vi "ziModGetNextNode.vi"(8 "Error In":errorcluster, 11 "ModHandle In":T5 {"ModHandle" format="0x%08x"; "Conn" format="0x%08x"}) -> (0 "Error Out":errorcluster, 2 "ModResults":T1, 3 "ModHandle Out":T5 {"ModHandle" format="0x%08x"; "Conn" format="0x%08x"}, 4 "NoData":bool)   [LabVIEW 2016, in "Zurich Instruments LabOne.lvlib"]
doc: "Use this device to extract the data from subscribed node, which you polled from device by ziModExecute.vi (with modal is false) or the ziModRead.vi. This allows to iterate through ModResults and return the <b>Path, the ValueType and the NoOfResults</b>. If this iterator, does not find any more data, the <b>NoData</b> flag is raised."
uses:
  Zurich Instruments LabOne.lvlib
  ziTypeModHandle.ctl
  ziTypeModResults.ctl
  Data/ziTypePollType.ctl
  ziTypeModSWTriggerHeader.ctl
  ziTypeModSweeperHeader.ctl
  ziModGetSWTriggerHeader.vi
  ziModGetSweeperHeader.vi
  Private/ziLV64.dll
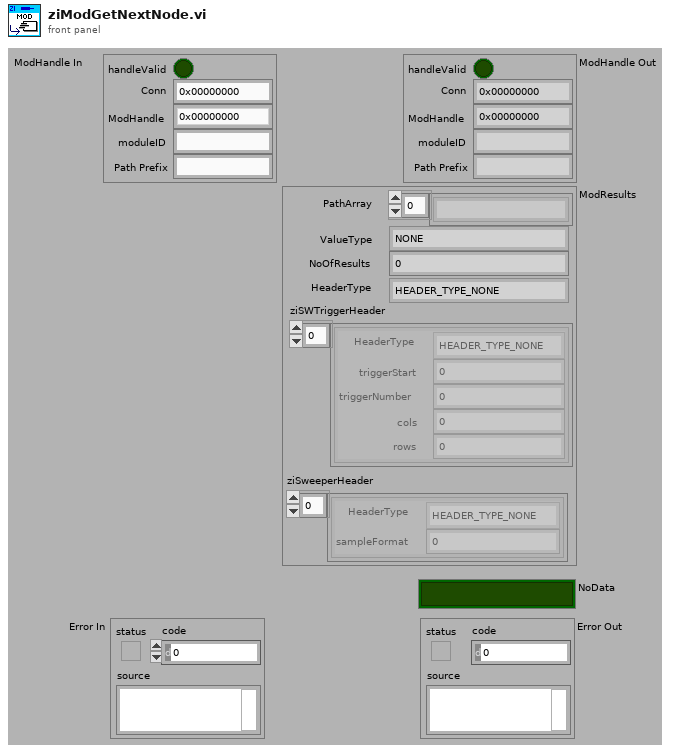
[diagram p1: front panel]
types:
  T1 = typedef "Zurich Instruments LabOne.lvlib/ziTypeModResults.ctl" = cluster{"PathArray":string[], "ValueType":T2, "NoOfResults":u64, "HeaderType":enum16{"HEADER_TYPE_NONE", "HEADER_TYPE_SWTRIGGER", "HEADER_TYPE_SWEEPER"}, "ziSWTriggerHeader":T3[], "ziSweeperHeader":T4[]}
  T2 = typedef "Zurich Instruments LabOne.lvlib/ziTypePollType.ctl" = enum16{"NONE", "DOUBLE_DATA", "INTEGER_DATA", "DEMOD_SAMPLE", "SCOPE_WAVE_HF2", "AUXIN_SAMPLE", "DIO_SAMPLE", "BYTE_ARRAY", "PWA_WAVE", "9", "10", "11", "12", "13", "14", "15", "TREE_CHANGE_DEPRI", "17", "ERROR", "19", "20", "21", "22", "23", "24", "25", "26", "27", "28", "29", "30", "31", "DOUBLE_DATA_TS", "INTEGER_DATA_TS", "34", "SCOPE_WAVE", "36", "37", "BYTE_ARRAY_TS", "39", "40", "41", "42", "43", "44", "45", "CNT_DATA", "47", "TREE_CHANGE", "49", "50", "51", "52", "53", "54", "55", "56", "57", "58", "59", "60", "61", "62", "63", "SWEEPER_DATA", "SPECTRUM_DATA", "ADVISOR_DATA", "67", "IMP_DATA"}
  T3 = typedef "Zurich Instruments LabOne.lvlib/ziTypeModSWTriggerHeader.ctl" = cluster{"HeaderType":enum8{"HEADER_TYPE_NONE", "HEADER_TYPE_SWTRIGGER", "HEADER_TYPE_SWEEPER"}, "triggerStart":u64, "triggerNumber":u64, "cols":u32, "rows":u32}
  T4 = typedef "Zurich Instruments LabOne.lvlib/ziTypeModSweeperHeader.ctl" = cluster{"HeaderType":enum8{"HEADER_TYPE_NONE", "HEADER_TYPE_SWTRIGGER", "HEADER_TYPE_SWEEPER"}, "sampleFormat":u8}
  T5 = typedef "Zurich Instruments LabOne.lvlib/ziTypeModHandle.ctl" = cluster{"handleValid":bool, "Conn":u64, "ModHandle":u64, "moduleID":string, "Path Prefix":string}
  T6 = enum16{"HEADER_TYPE_NONE", "HEADER_TYPE_SWTRIGGER", "HEADER_TYPE_SWEEPER"}
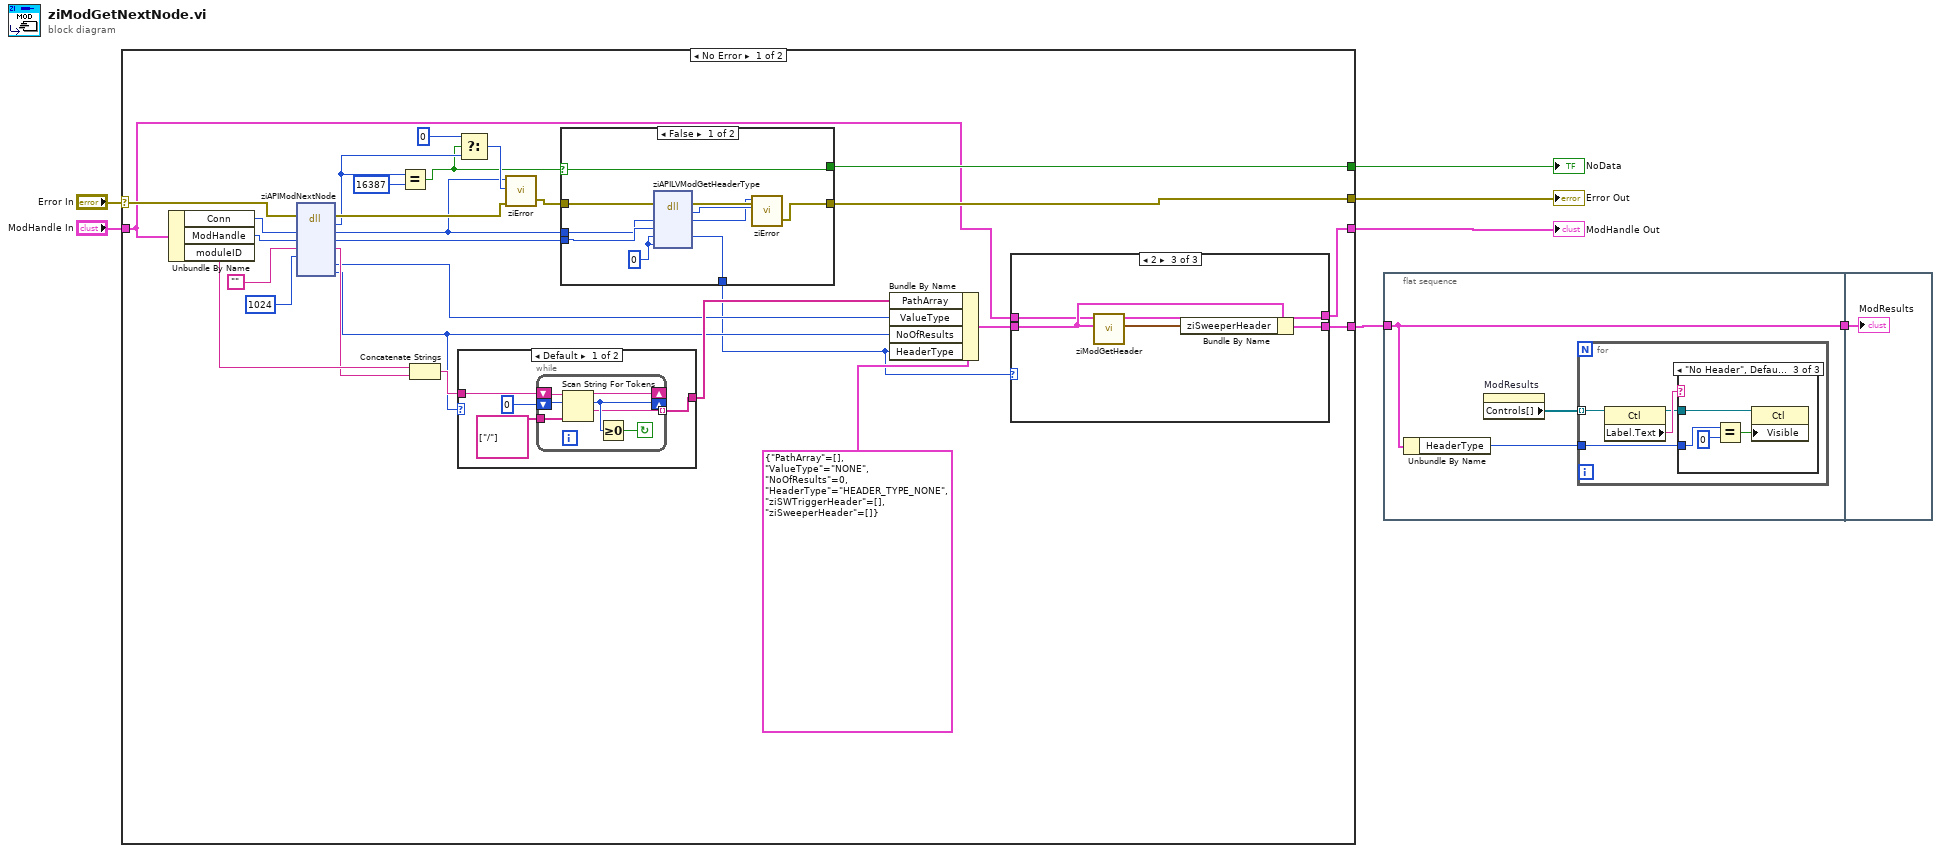
[diagram p0: block diagram]
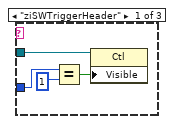
[diagram p2: hidden frame]
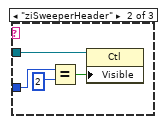
[diagram p3: hidden frame]
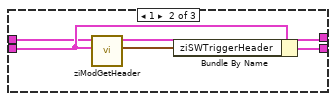
[diagram p5: hidden frame]
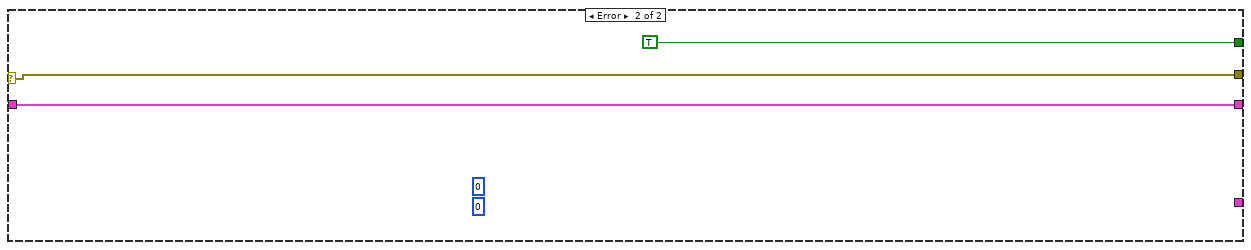
[diagram p8: hidden frame]
diagram:
  n1 = case shown="No Error" "Error In" {
    selector: "Error In" -> [w33 w71]
    tunnel: [w21 w71] -> w3
    tunnel: [w9 w73] -> w4
    tunnel: "ModHandle In" -> [w10 w73]
    tunnel: [w18 TRUE] -> w5
    tunnel: [w11 _] -> w2
    frame No Error {
      n2 = Unbundle By Name(w10) -> ("Conn"=w35:u64, "ModHandle"=w34:u64, "moduleID"=w25:string)
      n3 = dll-call lib="C:/Users/putkonen.CPFS/Desktop/resonant_ultrasound_arxiv/maglab ultrasound -- arkady --arxiv/Zurich/Zurich Instruments/LabOne/API/LabVIEW/Zurich Instruments LabOne/Private/ziLV*.*" fn="ziAPIModNextNode"(error in=w33, "Conn"=w35, "ModHandle"=w34, "Path"="", "bufferSize"=u32 1024) -> (error out=w32:errorcluster, "return type"=w28:u32, "Conn"=w17:u64, "ModHandle"=w22:u64, "Path"=w24:string, "valueType"=w14:u64, "NoOfResults"=w15:u64)  [unwired: 5 in, 1 out]
      n4 = Equal?(x=w28, y=u32 16387) -> (x = y?=w19:bool)
      n5 = Concatenate Strings(w25, w24) -> (w23:string)
      n6 = case shown="Default" w15 {
        tunnel: w23 -> [w61 _]
        tunnel: [w62 _] -> w16
        frame Default {
          n7 = while {
            shift-right: [w68] -> _
            shift-left: w61 -> [w70]
            shift-right: [w67] -> _
            shift-left: 0 ("offset past token") -> [w69]
            tunnel: [w65] -> w62 mode=indexing
            tunnel: string[] ["/"] ("delimiters (\\s,\\t,\\r,\\n)") -> [w64]
            stop <- w66 continue-if-true
            n8 = Scan String For Tokens(6:w64, 8:w69, 9:w70) -> (1:w65:string, 2:w67:i32, 3:w68:string)  [unwired: 1 in, 3 out]
            n9 = Greater Or Equal To 0?(x=w67) -> (x >= 0?=w66:bool)
          }
        }
        frame 0 {
        }
      }
      n10 = Select(t=u32 0, s=w19, f=w28) -> (s? t:f=w26:u32)
      n11 = call "ziError.vi"("Conn"=w17, "ziErrorCode"=w26, "Error In"=w32) -> ("Error Out"=w20:errorcluster)  [unwired: 2 in, 1 out]
      n12 = case shown="False" w19 {
        selector: w19 -> [w53 w58]
        tunnel: w22 -> [w57 _]
        tunnel: w17 -> [w56 _]
        tunnel: [w55 w59] -> w21
        tunnel: w20 -> [w54 w59]
        tunnel: [w53 w58] -> w18
        tunnel: [w48 _] -> w8
        frame False {
          w52 = u64 0 ("chunk_idx")
          n13 = dll-call lib="C:/Users/putkonen.CPFS/Desktop/resonant_ultrasound_arxiv/maglab ultrasound -- arkady --arxiv/Zurich/Zurich Instruments/LabOne/API/LabVIEW/Zurich Instruments LabOne/Private/ziLV*.*" fn="ziAPILVModGetHeaderType"(error in=w54, "Conn"=w56, "ModHandle"=w57, "headertype"=w52, "chunk_idx"=w52) -> (error out=w50:errorcluster, "return type"=w51:u32, "Conn"=w49:u64, "headertype"=w48:u8)  [unwired: 4 in, 1 out]
          n14 = call "ziError.vi"("Conn"=w49, "ziErrorCode"=w51, "Error In"=w50) -> ("Error Out"=w55:errorcluster)  [unwired: 2 in, 1 out]
        }
        frame True {
        }
      }
      n15 = Bundle By Name "Bundle By Name"(cluster=T1 {"PathArray"=[], "ValueType"=enum."NONE", "NoOfResults"=0, "HeaderType"=enum."HEADER_TYPE_NONE", "ziSWTriggerHeader"=[], "ziSweeperHeader"=[]} ("ziModResults 2"), "PathArray"=w16, "ValueType"=w14, "NoOfResults"=w15, "HeaderType"=w8) -> (w12:T1)
      n16 = case shown="2" w8 {
        tunnel: w12 -> [w37 w42 w47]
        tunnel: [w37 w41 w46] -> w11
        tunnel: w10 -> [w36 w40 w45]
        tunnel: [w36 w39 w44] -> w9
        frame 0, Default {
        }
        frame 1 {
          n17 = call-poly "ziModGetHeader.vi"("ModResults"=w42, "ModHandle In"=w40) -> ("SWTriggerHeader"=w38:T3[], "ModHandle Out"=w39:T5)  [unwired: 7 in, 1 out]
          n18 = Bundle By Name "Bundle By Name"(cluster=w42, "ziSWTriggerHeader"=w38) -> (w41:T1)
        }
        frame 2 {
          n19 = call-poly "ziModGetHeader.vi"("ModResults"=w47, "ModHandle In"=w45) -> ("SweeperHeader"=w43:T4[], "ModHandle Out"=w44:T5)  [unwired: 7 in, 1 out]
          n20 = Bundle By Name "Bundle By Name"(cluster=w47, "ziSweeperHeader"=w43) -> (w46:T1)
        }
      }
    }
    frame Error {
      (unwired) u64 0 ("NoOfResults")
      (unwired) u64 0 ("valueType")
    }
  }
  "Error Out" <- w3
  "ModHandle Out" <- w4
  "NoData" <- w5
  n21 = flat-sequence {
    tunnel: w2 -> [w75]
    tunnel: [w75] -> w1
    tunnel: w1 -> [w93]
    frame #0 {
      n22 = Unbundle By Name(w75) -> ("HeaderType"=w74:T6)
      n23 = property on="ModResults" class="Clust (strict)"() -> ("Controls[]"=w76:refnum<vi>[])  [unwired: 2 in, 2 out]
      n24 = for {
        tunnel: w76 -> [w80] mode=indexing
        tunnel: w74 -> [w77]
        n25 = property class="Ctl"(reference=w80) -> (reference out=w78:refnum<vi>, "Label.Text"=w79:string)  [unwired: 1 in, 1 out]
        n26 = case shown="\"No Header\", Default" w79 {
          tunnel: w78 -> [w84 w88 w92]
          tunnel: w77 -> [w83 w87 w91]
          frame "ziSWTriggerHeader" {
            n27 = Equal?(x=w83, y=u8 1) -> (x = y?=w82:bool)
            n28 = property class="Ctl"(reference=w84, "Visible"=w82) -> ()  [unwired: 1 in, 2 out]
          }
          frame "ziSweeperHeader" {
            n29 = Equal?(x=w87, y=u8 2) -> (x = y?=w86:bool)
            n30 = property class="Ctl"(reference=w88, "Visible"=w86) -> ()  [unwired: 1 in, 2 out]
          }
          frame "No Header", Default {
            n31 = Equal?(x=w91, y=u8 0) -> (x = y?=w90:bool)
            n32 = property class="Ctl"(reference=w92, "Visible"=w90) -> ()  [unwired: 1 in, 2 out]
          }
        }
      }
    }
    frame #1 {
      "ModResults" <- w93
    }
  }
